vi "replaceTypedefWithItemFromNewLibrary.vi"(6 "Typedef VI Reference":refnum<vi>, 8 "error in (no error)":errorcluster, 9 "specific class reference":refnum<vi>, 10 "Calling VI Reference":refnum<vi>, 11 "Constant in":refnum<class "Constant.lvclass">) -> (0 "error out":errorcluster, 3 "Constant out":refnum<class "Constant.lvclass">)   [LabVIEW 2016, in "Constant.lvclass"]
uses:
  Constant.lvclass
  C:/LSST_TS/SystemSW/ct_tools/GObject/GObject.lvclass
  GObject/GObject.lvclass/GObject.ctl
  Search/Search.lvclass/Search.ctl
  Variables/CtlsReplaced.vi
  Variables/CtlsReplaceFailed.vi
  Search/Search.lvclass
  Variables/SwitchDependenciesVariables.lvlib
  GObject/GObject.lvclass
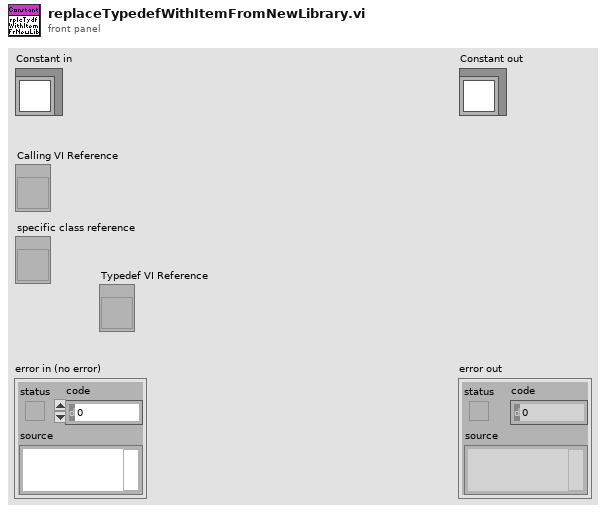
[diagram p1: front panel]
types:
  T1 = typedef "LibraryMemberNameReplacement.ctl" = cluster{"String To Replace in VI names":string, "String To Replace in Control names":string, "New String in VI names":string, "New String in Control names":string}
  T2 = typedef "LibraryDirectories.ctl" = cluster{"OldLibraryDirectory":string, "NewLibraryDirectory":string}
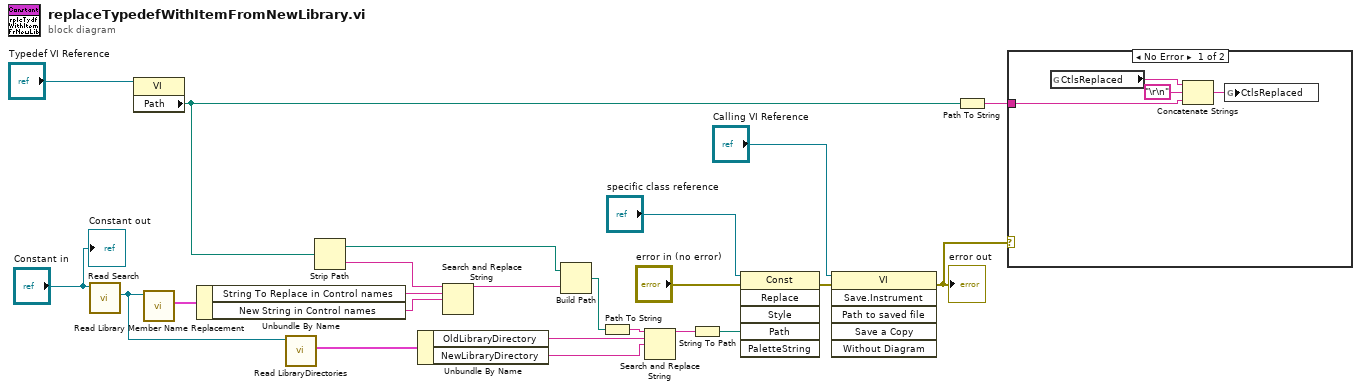
[diagram p0: block diagram]
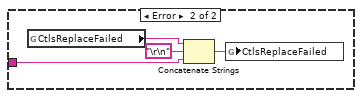
[diagram p2: hidden frame]
diagram:
  n1 = call "Read Search.vi"("DiagramObject in"="Constant in") -> ("Search.lvclass"=w7:refnum<class "Search.lvclass">)  [unwired: 9 in, 1 out]
  n2 = property class="VI"(reference="Typedef VI Reference") -> ("Path"=w1:path)  [unwired: 1 in, 2 out]
  n3 = call "Read Library Member Name Replacement.vi"("ProjectItem in"=w7) -> ("Library Member Name Replacement"=w9:T1)  [unwired: 9 in, 1 out]
  n4 = Unbundle By Name(w9) -> ("String To Replace in Control names"=w19:string, "New String in Control names"=w18:string)
  n5 = call "Read LibraryDirectories.vi"("ProjectItem in"=w7) -> ("LibraryDirectories"=w10:T2)  [unwired: 9 in, 1 out]
  n6 = Strip Path(path=w1) -> (stripped path=w17:path, name=w20:string)
  n7 = Unbundle By Name(w10) -> ("OldLibraryDirectory"=w12:string, "NewLibraryDirectory"=w11:string)
  n8 = Search and Replace String(input string=w20, search string=w19, replace string=w18) -> (result string=w16:string)  [unwired: 5 in, 3 out]
  n9 = Build Path(base path=w17, name or relative path=w16) -> (appended path=w15:path)
  n10 = Path To String(path=w15) -> (string=w14:string)
  n11 = Search and Replace String(input string=w14, search string=w12, replace string=w11) -> (result string=w13:string)  [unwired: 5 in, 3 out]
  n12 = String To Path(string=w13) -> (path=w23:path)
  n13 = invoke class="Const" method="Replace"(reference="specific class reference", error in="error in (no error)", "Path"=w23) -> (error out=w21:errorcluster)  [unwired: 3 in, 5 out]
  n14 = invoke class="VI" method="Save.Instrument"(reference="Calling VI Reference", error in=w21) -> (error out=w5:errorcluster)  [unwired: 4 in, 5 out]
  "error out" <- w5
  n15 = Path To String(path=w1) -> (string=w8:string)
  n16 = case shown="No Error" w5 {
    tunnel: w8 -> [w25 w29]
    frame No Error {
      n17 = global read "CtlsReplaced.vi" "CtlsReplaced"() -> (w27:string)
      n18 = Concatenate Strings(w27, "\r\n", w25) -> (w24:string)
      n19 = global write "CtlsReplaced.vi" "CtlsReplaced"(w24) -> ()
    }
    frame Error {
      n20 = global read "CtlsReplaceFailed.vi" "CtlsReplaceFailed"() -> (w31:string)
      n21 = Concatenate Strings(w31, "\r\n", w29) -> (w28:string)
      n22 = global write "CtlsReplaceFailed.vi" "CtlsReplaceFailed"(w28) -> ()
    }
  }
  "Constant out" <- "Constant in"
